vi "Example - Multipart File Upload.vi"() -> ()   [LabVIEW 2020]
uses:
  MultipartForm.lvclass
  ClientBuilder/ClientBuilder.lvclass
  Client/Client.lvclass
  Request/Request.lvclass
  Headers/Headers.lvclass
panel:
  in  "file_name":string="file"
  in  "field_value":string="Test file upload"
  in  "field_name":string="description"
  in  "file_path":path
  out "response_headers":cluster{"name":string, "value":string}[](array[cluster])
  out "response_body":string
  in  "url":string="https://httpbin.org/post"
  in  "Abort":bool
  out "bytes received":u64
  out "total bytes":u64
  out "progress":dbl(slide) scale=0.0..100.0
  out "total (ms)":dbl
  in  "Start":bool
  in  "Exit":bool
  out "sending":bool
  # "0. Leave all default values alone\n1. Choose a file to upload (via \"file_path\" control)\n2. Press \"Start\" to upload it"
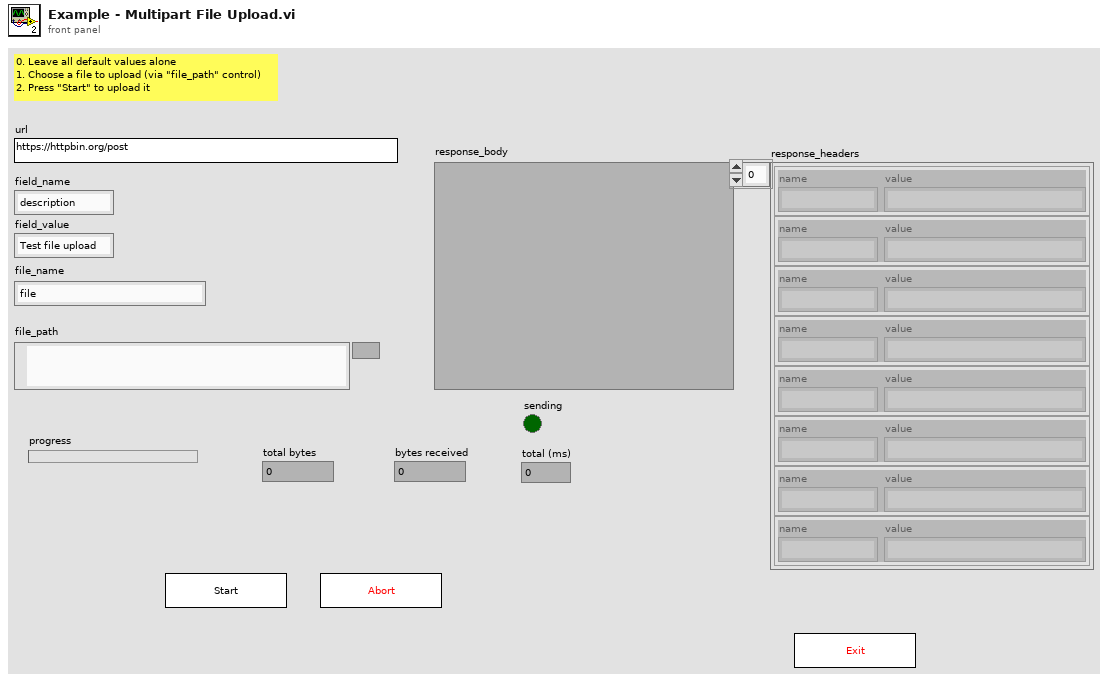
[diagram p1: front panel]
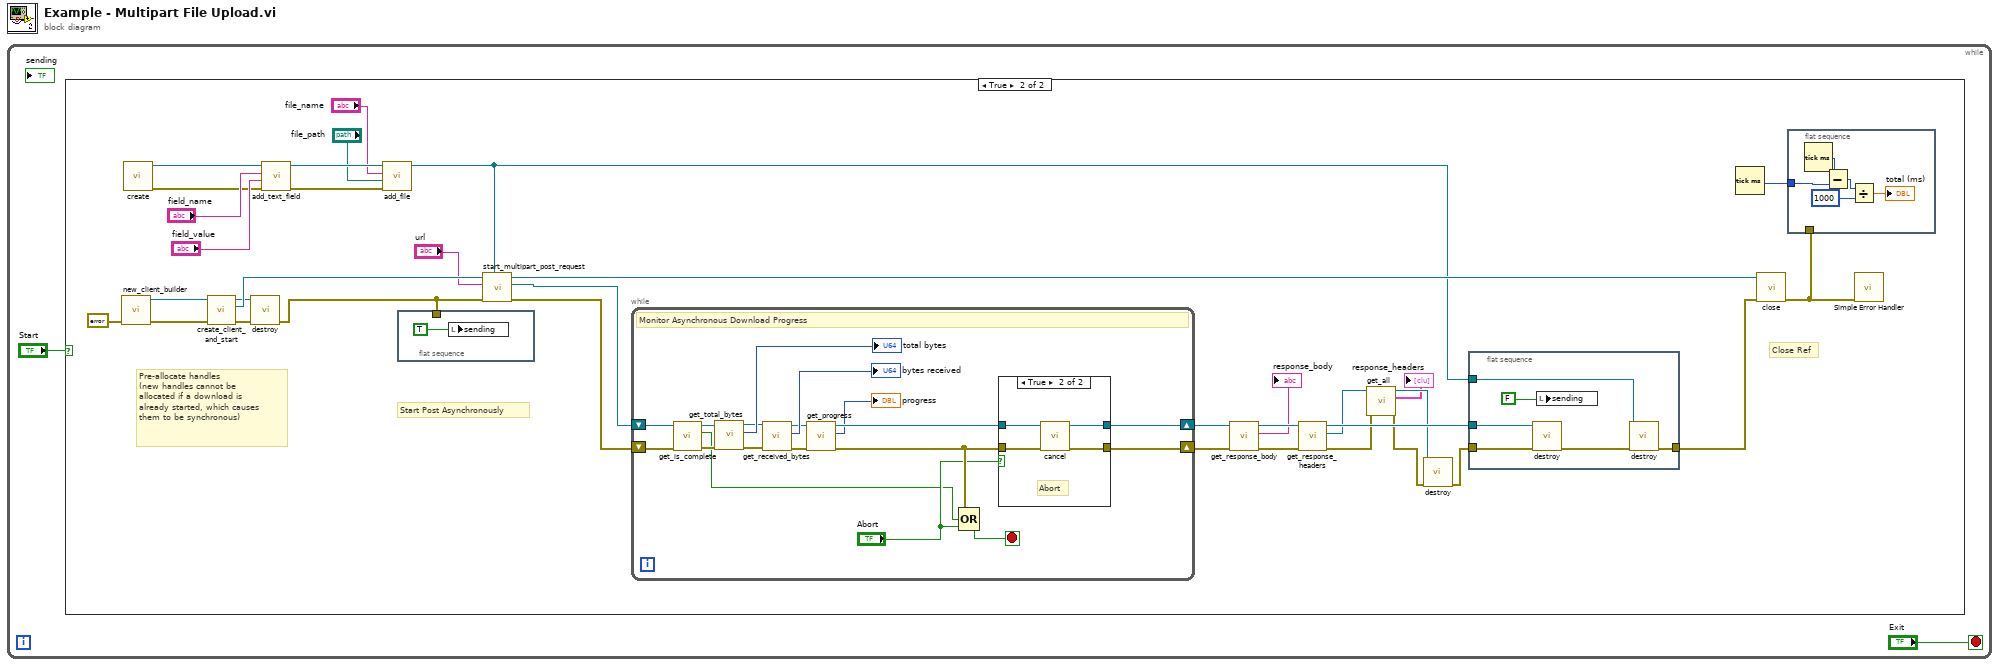
[diagram p0: block diagram]
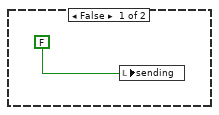
[diagram p2: hidden frame]
diagram:
  n1 = while {
    stop <- "Exit" stop-if-true
    n2 = case shown="True" "Start" {
      frame False {
        n3 = local write "sending"(FALSE ("downloading")) -> ()
      }
      frame True {
        # "Start Post Asynchronously"
        # "Close Ref"
        # "Pre-allocate handles\n(new handles cannot be allocated if a download is already started, which causes them to be synchronous)"
        n4 = call "new_client_builder.vi"("error in (no error)"=errorcluster {"status"=FALSE, "code"=0, "source"=""} ("error out")) -> ("error out"=w32:errorcluster, "Client out"=w33:refnum<class "ClientBuilder.lvclass">)  [unwired: 9 in]
        n5 = call "create.vi"() -> ("error out"=w25:errorcluster, "MultipartForm out"=w24:refnum<class "MultipartForm.lvclass">)  [unwired: 10 in]
        n6 = call "create_client_and_start.vi"("error in"=w32, "ClientBuilder in"=w33) -> ("error out"=w28:errorcluster, "Client out"=w31:refnum<class "Client.lvclass">, "ClientBuilder out"=w29:refnum<class "ClientBuilder.lvclass">)  [unwired: 7 in]
        n7 = call "destroy.vi"("error in (no error)"=w28, "ClientBuilder in"=w29) -> ("error out"=w21:errorcluster)  [unwired: 9 in]
        n8 = call "add_text_field.vi"("error in"=w25, "field_value"="field_value", "field_name"="field_name", "MultipartForm in"=w24) -> ("error out"=w6:errorcluster, "MultipartForm out"=w8:refnum<class "MultipartForm.lvclass">)  [unwired: 5 in, 1 out]
        n9 = call "add_file.vi"("error in"=w6, "file_path"="file_path", "name"="file_name", "MultipartForm in"=w8) -> ("MultipartForm out"=w7:refnum<class "MultipartForm.lvclass">)  [unwired: 6 in, 1 out]
        n10 = flat-sequence {
          tunnel: w21 -> [_]
          frame #0 {
            n11 = local write "sending"(TRUE ("downloading")) -> ()
          }
        }
        n12 = call "start_multipart_post_request.vi"("MultipartForm"=w7, "error in (no error)"=w21, "url"="url", "Client in"=w31) -> ("error out"=w38:errorcluster, "Request"=w37:refnum<class "Request.lvclass">, "Client out"=w36:refnum<class "Client.lvclass">)  [unwired: 5 in]
        n13 = while {
          shift-right: [w65] -> w19
          shift-left: w38 -> [w66]
          shift-right: [w52] -> w17
          shift-left: w37 -> [w67]
          stop <- w68 stop-if-true
          # "Monitor Asynchronous Download Progress"
          n14 = call "get_is_complete.vi"("error in (no error)"=w66, "Request in"=w67) -> ("error out"=w53:errorcluster, "is_complete"=w51:bool, "Request out"=w56:refnum<class "Request.lvclass">)  [unwired: 7 in]
          n15 = call "get_total_bytes.vi"("error in (no error)"=w53, "Request in"=w56) -> ("error out"=w54:errorcluster, "total_bytes"=→"total bytes":u64, "Request out"=w55:refnum<class "Request.lvclass">)  [unwired: 7 in]
          n16 = call "get_received_bytes.vi"("error in (no error)"=w54, "Request in"=w55) -> ("error out"=w57:errorcluster, "received_bytes"=→"bytes received":u64, "Request out"=w58:refnum<class "Request.lvclass">)  [unwired: 7 in]
          n17 = call "get_progress.vi"("error in (no error)"=w57, "Request in"=w58) -> ("error out"=w64:errorcluster, "progress"=→"progress":i32, "Request out"=w62:refnum<class "Request.lvclass">)  [unwired: 7 in]
          n18 = Compound Arithmetic op=OR(w64, w51, "Abort") -> (w68:bool)
          n19 = case shown="True" "Abort" {
            tunnel: [w70 w74] -> w65
            tunnel: w64 -> [w70 w73]
            tunnel: w62 -> [w69 w72]
            tunnel: [w69 w71] -> w52
            frame False {
            }
            frame True {
              # "Abort"
              n20 = call "cancel.vi"("error in (no error)"=w73, "Request in"=w72) -> ("error out"=w74:errorcluster, "Request out"=w71:refnum<class "Request.lvclass">)  [unwired: 7 in, 1 out]
            }
          }
        }
        n21 = call "get_response_body.vi"("error in (no error)"=w19, "Request in"=w17) -> ("error out"=w18:errorcluster, "string_value"=→"response_body":string, "Request in"=w16:refnum<class "Request.lvclass">)  [unwired: 7 in]
        n22 = call "get_response_headers.vi"("error in (no error)"=w18, "Request in"=w16) -> ("error out"=w11:errorcluster, "response_headers"=w13:refnum<class "Headers.lvclass">, "Request in"=w20:refnum<class "Request.lvclass">)  [unwired: 7 in]
        n23 = call "get_all.vi"("error in (no error)"=w11, "Headers in"=w13) -> ("error out"=w10:errorcluster, "headers"=→"response_headers":cluster{"name":string, "value":string}[], "Headers in"=w12:refnum<class "Headers.lvclass">)  [unwired: 6 in, 1 out]
        n24 = call "destroy.vi"("error in (no error)"=w10, "Headers in"=w12) -> ("error out"=w14:errorcluster)  [unwired: 9 in]
        n25 = flat-sequence {
          tunnel: w20 -> [w45]
          tunnel: w14 -> [w44]
          tunnel: w7 -> [w43]
          tunnel: [w41] -> w23
          frame #0 {
            n26 = call "destroy.vi"("error in (no error)"=w44, "Request in"=w45) -> ("error out"=w42:errorcluster)  [unwired: 8 in, 1 out]
            n27 = local write "sending"(FALSE ("downloading")) -> ()
            n28 = call "destroy.vi"("error in (no error)"=w42, "MultipartForm in"=w43) -> ("error out"=w41:errorcluster)  [unwired: 9 in]
          }
        }
        n29 = Tick Count (ms)() -> (millisecond timer value=w34:u32)
        n30 = call "close.vi"("error in (no error)"=w23, "Client in"=w36) -> ("error out"=w35:errorcluster)  [unwired: 9 in]
        n31 = flat-sequence {
          tunnel: w35 -> [_]
          tunnel: w34 -> [w49]
          frame #0 {
            n32 = Tick Count (ms)() -> (millisecond timer value=w50:u32)
            n33 = Subtract(x=w50, y=w49) -> (x-y=w48:u32)
            n34 = Divide(x=w48, y=u32 1000) -> (x/y=→"total (ms)":dbl)
          }
        }
        n35 = call <vilib>:"Simple Error Handler.vi"("error in (no error)"=w35) -> ()  [unwired: 4 in, 5 out]
      }
    }
  }
